vi "prop power.vi"(9 "Control Parameters":T1 {"Settle time" format="%.2f"; "Derivative time" format="%.2f"; "Integral time" format="%.2f"; "Settle bandwidth" format="%.2f"; "Control bandwidth" format="%.2f"; "Setpoint" format="%.2f"}, 10 "Temp In (deg C)":dbl) -> (3 "p out":dbl)   [LabVIEW 2011]
uses:
  P350 W12 content master/Assignments/P5 T 2-28 to T 3-6/P5 sim start/typedefs/control parameters.ctl
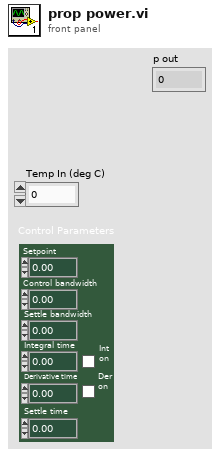
[diagram p1: front panel]
types:
  T1 = typedef "control parameters.ctl" = cluster{"Setpoint":dbl, "Control bandwidth":dbl, "Settle bandwidth":dbl, "Integral time":dbl, "Int\non":bool, "Derivative time":dbl, "Der\non":bool, "Settle time":dbl}
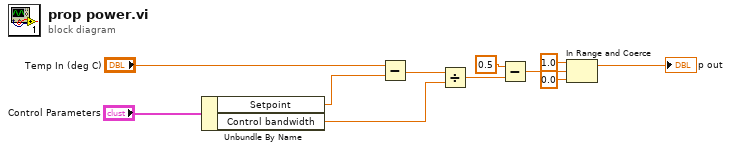
[diagram p0: block diagram]
diagram:
  n1 = Unbundle By Name("Control Parameters") -> ("Setpoint"=w9:dbl, "Control bandwidth"=w8:dbl)
  n2 = Subtract(x="Temp In (deg C)", y=w9) -> (x-y=w7:dbl)
  n3 = Divide(x=w7, y=w8) -> (x/y=w6:dbl)
  n4 = Subtract(x=0.5, y=w6) -> (x-y=w4:dbl)
  n5 = In Range and Coerce(upper limit=1.0, x=w4, lower limit=0.0) -> (coerced(x)=→"p out":dbl)  [unwired: 1 out]
